vi "IO参数设置.vi"(8 "布尔文本.文本":string, 9 "section (optional)":string, 10 "监测项描述":string) -> (2 "增加？":bool, 3 "簇1输出":T1)   [LabVIEW 2016, in "环境动力监测库.lvlib"]
uses:
  <vilib>/Utility/miscctls.llb/LVPointTypeDef.ctl
  <vilib>/Utility/config.llb/NI_LVConfig.lvlib
panel:
  in  "模拟量配置":bool
  in  "传感器型号:":enum16{"PLC", "ZLAN"}(ring)
  in  "簇1输入":T1
  in  "返回":bool
  in  "增加":bool
  in  "告警参数:":enum32{"禁用告警", "闭合告警", "断开告警"}(radio)
  in  "端口:":T2(ring)
  in  "监测项描述:":string
  # "基本设置"
  # "如:红外XX"
  # "传感器选择"
  # "端口选择"
  # "参数设置"
  # "告警方式选择"
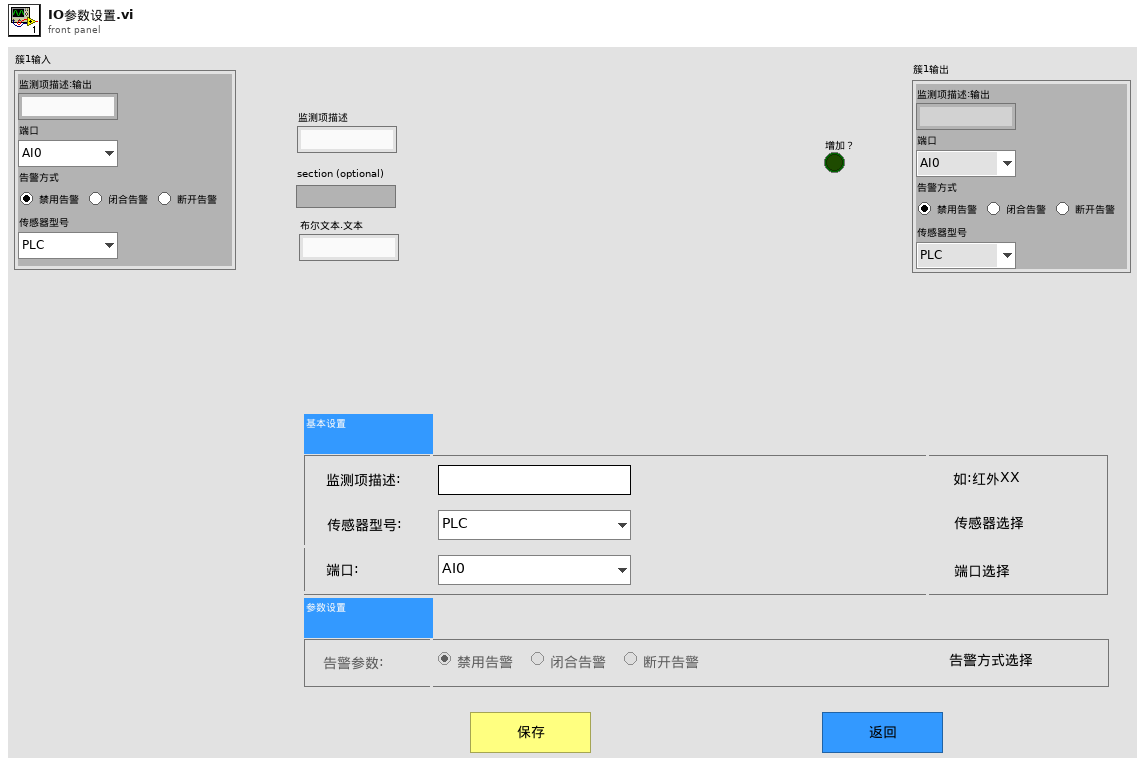
[diagram p1: front panel]
types:
  T1 = cluster{"监测项描述:输出":string, "端口":enum16{"AI0", "AI1", "AI2", "AI3", "AI4", "DI0", "DI1", "DI2", "DI3", "DI4", "DO0", "DO1", "DO2", "DO3", "DO4", "X0", "X1", "X2", "X3", "X4", "X5", "X6", "X7", "X8", "X9"}, "告警方式":enum32{"禁用告警", "闭合告警", "断开告警"}, "传感器型号":enum16{"PLC", "ZLAN"}}
  T2 = enum16{"AI0", "AI1", "AI2", "AI3", "AI4", "DI0", "DI1", "DI2", "DI3", "DI4", "DO0", "DO1", "DO2", "DO3", "DO4", "X0", "X1", "X2", "X3", "X4", "X5", "X6", "X7", "X8", "X9"}
  T3 = cluster{"模板选择:":enum16{"定时简报", "无(不告警)", "通用声光告警", "通用语言告警", "通用短信告警", "通用电话告警", "通用邮件告警", "通用声光+语音+短信告警", "通用声光+短信+电话告警", "通用多方式告警", "通用全方式告警", "自动按类型", "非告警时段", "自定义"}, "预警保持时间\n(s):":i16, "重复告警时间\n(s):":i16, "告警发送方式:":cluster{"声光":bool, "语音":bool, "短信":bool, "彩信":bool, "电话":bool, "邮件":bool, "联动1":bool, "联动2":bool}, "告警时段选择:":enum16{"全时段告警", "工作日告警", "周六周日告警", "非告警时段", "自定义"}, "告警抓拍设置:":enum16{"无"}, "告警短信内容:":string, "告警电话内容:":string, "告警解除方式:":cluster{"声光":bool, "语音":bool, "短信":bool, "彩信":bool, "电话":bool, "邮件":bool, "联动1":bool, "联动2":bool}, "告警解除内容:":string, "信息接收人:":cluster{"管理员":bool, "普通用户":bool}}
  T4 = typedef "LVPointTypeDef.ctl" = cluster{"Horizontal":i16, "Vertical":i16}
  T5 = typedef "NI_LVConfig.lvlib/Config Data RefNum.ctl" = refnum<k1>
  T6 = enum8{"Enabled", "Disabled", "Disabled and Grayed Out"}
  T7 = cluster{"漏水监测配置":cluster{"监测项描述:输出":string, "端口:":enum16{"AI0", "AI1", "AI2", "AI3", "AI4", "DI0", "DI1", "DI2", "DI3", "DI4", "DO0", "DO1", "DO2", "DO3", "DO4", "X0", "X1", "X2", "X3", "X4", "X5", "X6", "X7", "X8", "X9"}, "告警参数:":enum32{"禁用告警", "闭合告警", "断开告警"}, "传感器型号:":enum16{"PLC", "ZLAN"}}, "门禁开关监测配置":cluster{"监测项描述:输出":string, "端口:":enum16{"AI0", "AI1", "AI2", "AI3", "AI4", "DI0", "DI1", "DI2", "DI3", "DI4", "DO0", "DO1", "DO2", "DO3", "DO4", "X0", "X1", "X2", "X3", "X4", "X5", "X6", "X7", "X8", "X9"}, "告警参数:":enum32{"禁用告警", "闭合告警", "断开告警"}, "传感器型号:":enum16{"PLC", "ZLAN"}}, "温湿度监测配置":cluster{"监测项描述:输出":string, "端口:":enum16{"AI0", "AI1", "AI2", "AI3", "AI4", "DI0", "DI1", "DI2", "DI3", "DI4", "DO0", "DO1", "DO2", "DO3", "DO4", "X0", "X1", "X2", "X3", "X4", "X5", "X6", "X7", "X8", "X9"}, "告警参数:":enum32{"禁用告警", "闭合告警", "断开告警"}, "传感器型号:":enum16{"PLC", "ZLAN"}}, "烟雾监测配置":cluster{"监测项描述:输出":string, "端口:":enum16{"AI0", "AI1", "AI2", "AI3", "AI4", "DI0", "DI1", "DI2", "DI3", "DI4", "DO0", "DO1", "DO2", "DO3", "DO4", "X0", "X1", "X2", "X3", "X4", "X5", "X6", "X7", "X8", "X9"}, "告警参数:":enum32{"禁用告警", "闭合告警", "断开告警"}, "传感器型号:":enum16{"PLC", "ZLAN"}}, "冰箱监测配置":cluster{"监测项描述:输出":string, "端口:":enum16{"AI0", "AI1", "AI2", "AI3", "AI4", "DI0", "DI1", "DI2", "DI3", "DI4", "DO0", "DO1", "DO2", "DO3", "DO4", "X0", "X1", "X2", "X3", "X4", "X5", "X6", "X7", "X8", "X9"}, "告警参数:":enum32{"禁用告警", "闭合告警", "断开告警"}, "传感器型号:":enum16{"PLC", "ZLAN"}}, "排气扇监测配置":cluster{"监测项描述:输出":string, "端口:":enum16{"AI0", "AI1", "AI2", "AI3", "AI4", "DI0", "DI1", "DI2", "DI3", "DI4", "DO0", "DO1", "DO2", "DO3", "DO4", "X0", "X1", "X2", "X3", "X4", "X5", "X6", "X7", "X8", "X9"}, "告警参数:":enum32{"禁用告警", "闭合告警", "断开告警"}, "传感器型号:":enum16{"PLC", "ZLAN"}}}
  T8 = cluster{"原始值最小值":dbl, "原始值最大值":dbl, "转换值最小值":dbl, "转换值最大值":dbl, "原始值最小值 2":dbl, "原始值最大值 2":dbl, "转换值最小值 2":dbl, "转换值最大值 2":dbl, "原始值最小值 3":dbl, "原始值最大值 3":dbl, "转换值最小值 3":dbl, "转换值最大值 3":dbl, "原始值最小值 4":dbl, "原始值最大值 4":dbl, "转换值最小值 4":dbl, "转换值最大值 4":dbl, "转换值最大值 5":dbl, "转换值最小值 5":dbl, "原始值最大值 5":dbl, "原始值最小值 5":dbl, "转换值最大值 6":dbl, "转换值最小值 6":dbl, "原始值最大值 6":dbl, "原始值最小值 6":dbl, "转换值最大值 7":dbl, "转换值最小值 7":dbl, "原始值最大值 7":dbl, "原始值最小值 7":dbl, "转换值最大值 8":dbl, "转换值最小值 8":dbl, "原始值最大值 8":dbl, "原始值最小值 8":dbl}
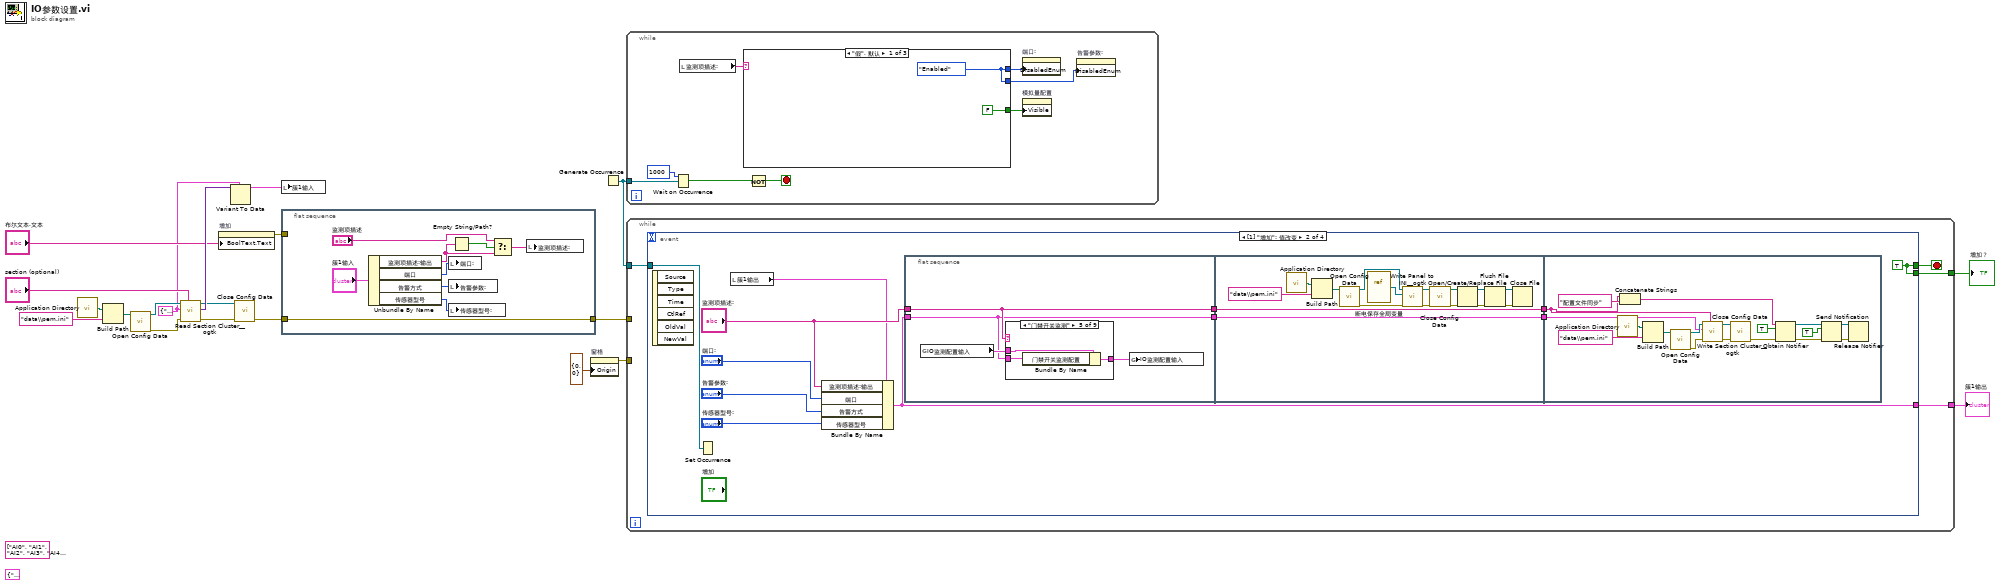
[diagram p0: block diagram]
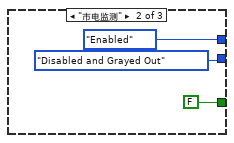
[diagram p2: hidden frame]
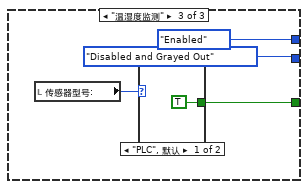
[diagram p3: hidden frame]
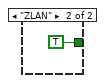
[diagram p4: hidden frame]
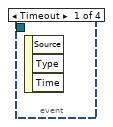
[diagram p5: hidden frame]
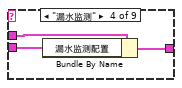
[diagram p9: hidden frame]
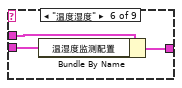
[diagram p10: hidden frame]
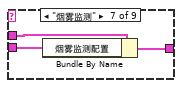
[diagram p11: hidden frame]
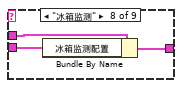
[diagram p12: hidden frame]
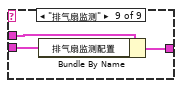
[diagram p13: hidden frame]
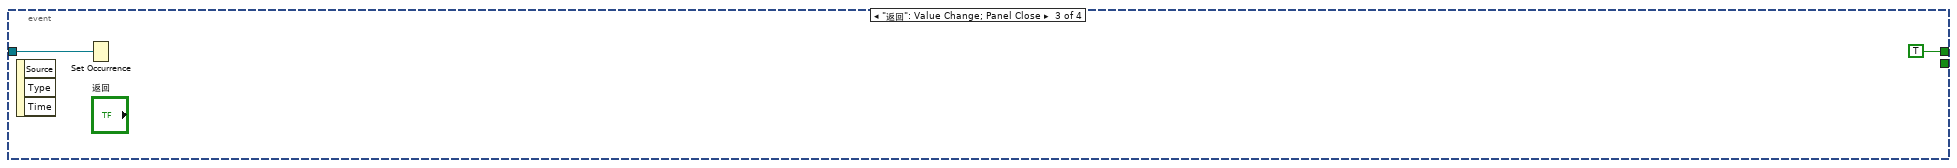
[diagram p14: hidden frame]
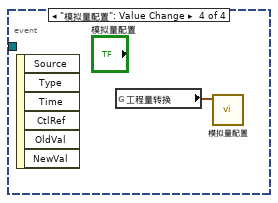
[diagram p15: hidden frame]
diagram:
  w1 = T1 {"监测项描述:输出"="", "端口"=enum."AI0", "告警方式"=enum."闭合告警", "传感器型号"=enum."PLC"} ("簇1输入")
  (unwired) string[] ["AI0", "AI1", "AI2", "AI3", "AI4", "DI0", "DI1", "DI2", "DI3", "DI4", "DO0", "DO1", "DO2", "DO3", "DO4", "X0", "X1", "X2", "X3", "X4", "X5", "X6", "X7", "X8", "X9"] ("字符串[]")
  (unwired) T3 {"模板选择:"=enum."定时简报", "预警保持时间\n(s):"=0, "重复告警时间\n(s):"=0, "告警发送方式:"={"声光"=FALSE, "语音"=FALSE, "短信"=FALSE, "彩信"=FALSE, "电话"=FALSE, "邮件"=FALSE, "联动1"=FALSE, "联动2"=FALSE}, "告警时段选择:"=enum."全时段告警", "告警抓拍设置:"=enum."无", "告警短信内容:"="", "告警电话内容:"="", "告警解除方式:"={"声光"=FALSE, "语音"=FALSE, "短信"=FALSE, "彩信"=FALSE, "电话"=FALSE, "邮件"=FALSE, "联动1"=FALSE, "联动2"=FALSE}, "告警解除内容:"="", "信息接收人:"={"管理员"=FALSE, "普通用户"=FALSE}} ("数据")
  n1 = call <vilib>:"Application Directory.vi"() -> ("Application Directory"=w14:path)
  n2 = Build Path(base path=w14, name or relative path="data\\pem.ini" ("名称或相对路径")) -> (appended path=w15:path)
  n3 = call <vilib>:"Open Config Data.vi"("configuration file path"=w15) -> ("error out"=w16:errorcluster, "refnum"=w17:T5)  [unwired: 8 in, 1 out]
  n4 = call <userlib>:"Read Section Cluster__ogtk.vi"("section (optional)"="section (optional)", "error in (no error)"=w16, "Section Formatted Cluster Type"=w1, "refnum"=w17) -> ("error out"=w4:errorcluster, "Section Formatted Cluster"=w11:variant, "dup refnum"=w5:T5)  [unwired: 3 in, 2 out]
  n5 = property on="增加" class="Bool"("BoolText.Text"="布尔文本.文本") -> (error out=w7:errorcluster)  [unwired: 2 in, 1 out]
  n6 = Variant To Data(type=w1, Variant=w11) -> (data=w6:T1)  [unwired: 1 in, 1 out]
  n7 = call <vilib>:"Close Config Data.vi"("error in (no error)"=w4, "refnum"=w5) -> ("error out"=w10:errorcluster)  [unwired: 8 in, 1 out]
  n8 = local write "簇1输入"(w6) -> ()
  n9 = flat-sequence {
    tunnel: w10 -> [w28]
    tunnel: [w28] -> w9
    tunnel: w7 -> [_]
    frame #0 {
      n10 = Unbundle By Name("簇1输入") -> ("监测项描述:输出"=w25:string, "端口"=w23:T2, "告警方式"=w22:enum32{"禁用告警", "闭合告警", "断开告警"}, "传感器型号"=w21:enum16{"PLC", "ZLAN"})
      n11 = local write "端口:"(w23) -> ()
      n12 = local write "告警参数:"(w22) -> ()
      n13 = local write "传感器型号:"(w21) -> ()
      n14 = Empty String/Path?(string/path=w25) -> (empty?=w27:bool)
      n15 = Select(t="监测项描述", s=w27, f=w25) -> (s? t:f=w24:string)
      n16 = local write "监测项描述:"(w24) -> ()
    }
  }
  n17 = property on="窗格" class="Pane"("Origin"=T4 {"Horizontal"=0, "Vertical"=0} ("原点")) -> (error out=w18:errorcluster)  [unwired: 2 in, 1 out]
  n18 = Generate Occurrence() -> (w3:refnum<k4>)
  n19 = while {
    tunnel: w3 -> [w35]
    stop <- w34 stop-if-true
    n20 = Wait on Occurrence(2:w35, 3:1000 ("毫秒超时(-1)")) -> (0:w36:bool)  [unwired: 1 in]
    n21 = local read "监测项描述:"() -> (w33:string)
    n22 = case shown="\"假\", 默认" w33 {
      tunnel: [FALSE ("可见") FALSE ("可见") w45] -> w32
      tunnel: [w38 T6."Enabled" ("禁用") T6."Enabled" ("禁用")] -> w31
      tunnel: [w38 T6."Disabled and Grayed Out" ("禁用") T6."Disabled and Grayed Out" ("禁用")] -> w30
      frame "假", Default {
        w38 = T6."Enabled" ("禁用")
      }
      frame "市电监测" {
      }
      frame "温湿度监测" {
        n23 = local read "传感器型号:"() -> (w46:enum16{"PLC", "ZLAN"})
        n24 = case shown="\"PLC\", 默认" w46 {
          tunnel: [TRUE ("可见") TRUE ("可见")] -> w45
          frame "PLC", Default {
          }
          frame "ZLAN" {
          }
        }
      }
    }
    n25 = Not(x=w36) -> (.not. x?=w34:bool)
    n26 = property on="端口:" class="Enum (严格)"("DisabledEnum"=w31) -> ()  [unwired: 2 in, 2 out]
    n27 = property on="模拟量配置" class="Bool"("Visible"=w32) -> ()  [unwired: 2 in, 2 out]
    n28 = property on="告警参数:" class="RadioBtnsControl (严格)"("DisabledEnum"=w30) -> ()  [unwired: 2 in, 2 out]
  }
  n29 = while {
    tunnel: [w52] -> w2
    tunnel: [w50] -> w20
    tunnel: w18 -> [_]
    tunnel: w9 -> [_]
    tunnel: w3 -> [w49]
    stop <- w51 stop-if-true
    n30 = event shown="[1] \"增加\": 值改变" {
      selector: _ -> [_ _ _ _]
      dyn-events: _ -> [_ _ _ _]
      timeout: _ -> [_ _ _ _]
      tunnel: [_ w64 TRUE _] -> w51
      tunnel: [_ w57 _ _] -> w52
      tunnel: [_ w64 _ _] -> w50
      tunnel: w49 -> [_ w62 w124 _]
      event Timeout {
        n31 = event-data() -> ()  [unwired: 1 in, 3 out]
      }
      event "增加": Value Change {
        w64 = TRUE
        n32 = event-data() -> ()  [unwired: 1 in, 6 out]
        n33 = Set Occurrence(w62) -> ()
        n34 = local read "簇1输出"() -> (w61:T1)
        n35 = Bundle By Name(cluster=w61, "监测项描述:输出"="监测项描述:", "端口"="端口:", "告警方式"="告警参数:", "传感器型号"="传感器型号:") -> (w57:T1)
        n36 = flat-sequence {
          tunnel: "监测项描述:" -> [w66]
          tunnel: w57 -> [w65]
          tunnel: [w66] -> w56
          tunnel: [w65] -> w54
          tunnel: w56 -> [w91]
          tunnel: [w91] -> w55
          tunnel: w54 -> [w90]
          tunnel: [w90] -> w53
          tunnel: w55 -> [w107]
          tunnel: w53 -> [w109]
          frame #0 {
            n37 = global read "断电保存全局变量.vi" "IO监测配置输入"() -> (w68:T7)
            n38 = case shown="\"门禁开关监测\"" w66 {
              tunnel: w68 -> [w69 w70 w71 w74 w77 w80 w83 w86 w89]
              tunnel: [w69 w70 w71 w73 w76 w79 w82 w85 w88] -> w67
              tunnel: w65 -> [_ _ _ w72 w75 w78 w81 w84 w87]
              frame "假", Default {
              }
              frame "市电监测" {
              }
              frame "空调监测" {
              }
              frame "漏水监测" {
                n39 = Bundle By Name(cluster=w74, "漏水监测配置"=w72) -> (w73:T7)
              }
              frame "门禁开关监测" {
                n40 = Bundle By Name(cluster=w77, "门禁开关监测配置"=w75) -> (w76:T7)
              }
              frame "温度湿度" {
                n41 = Bundle By Name(cluster=w80, "温湿度监测配置"=w78) -> (w79:T7)
              }
              frame "烟雾监测" {
                n42 = Bundle By Name(cluster=w83, "烟雾监测配置"=w81) -> (w82:T7)
              }
              frame "冰箱监测" {
                n43 = Bundle By Name(cluster=w86, "冰箱监测配置"=w84) -> (w85:T7)
              }
              frame "排气扇监测" {
                n44 = Bundle By Name(cluster=w89, "排气扇监测配置"=w87) -> (w88:T7)
              }
            }
            n45 = global write "断电保存全局变量.vi" "IO监测配置输入"(w67) -> ()
          }
          frame #1 {
            n46 = call <vilib>:"Application Directory.vi"() -> ("Application Directory"=w105:path)
            n47 = Build Path(base path=w105, name or relative path="data\\pem.ini" ("名称或相对路径")) -> (appended path=w103:path)
            n48 = call <vilib>:"Open Config Data.vi"("configuration file path"=w103) -> ("error out"=w101:errorcluster, "refnum"=w102:T5)  [unwired: 8 in, 1 out]
            n49 = vi-ref "断电保存全局变量.vi"() -> (w92:refnum<vi>)
            n50 = call <userlib>:"Write Panel to INI__ogtk.vi"("error in (no error)"=w101, "VI ref"=w92, "refnum"=w102) -> ("error out"=w99:errorcluster, "refnum out"=w100:T5)  [unwired: 7 in]
            n51 = call <vilib>:"Close Config Data.vi"("error in (no error)"=w99, "refnum"=w100) -> ("error out"=w93:errorcluster, "file path"=w94:path)  [unwired: 8 in]
            n52 = Open/Create/Replace File(file path (use dialog)=w94, error in=w93) -> (refnum out=w97:refnum<file>, error out=w98:errorcluster)  [unwired: 4 in, 1 out]
            n53 = Flush File(refnum=w97, error in=w98) -> (refnum out=w96:refnum<file>, error out=w95:errorcluster)
            n54 = Close File(refnum=w96, error in=w95) -> ()  [unwired: 2 out]
          }
          frame #2 {
            n55 = call <vilib>:"Application Directory.vi"() -> ("Application Directory"=w112:path)
            n56 = Concatenate Strings(w107, "配置文件同步" ("名称（未命名）")) -> (w106:string)
            n57 = Build Path(base path=w112, name or relative path="data\\pem.ini" ("名称或相对路径")) -> (appended path=w111:path)
            n58 = call <vilib>:"Open Config Data.vi"("configuration file path"=w111) -> ("error out"=w110:errorcluster, "refnum"=w123:T5)  [unwired: 8 in, 1 out]
            n59 = call <userlib>:"Write Section Cluster__ogtk.vi"("section (optional)"=w107, "error in (no error)"=w110, "Section Formatted Cluster"=w109, "refnum"=w123) -> ("error out"=w122:errorcluster, "dup refnum"=w121:T5)  [unwired: 6 in]
            n60 = call <vilib>:"Close Config Data.vi"("error in (no error)"=w122, "refnum"=w121) -> ("error out"=w118:errorcluster)  [unwired: 8 in, 1 out]
            n61 = Obtain Notifier(name (unnamed)=w106, notification data type=TRUE, error in (no error)=w118) -> (notifier out=w116:refnum<notifier>, error out=w117:errorcluster)  [unwired: 1 in, 1 out]
            n62 = Send Notification(notification=TRUE ("通知"), notifier=w116, error in (no error)=w117) -> (notifier out=w119:refnum<notifier>, error out=w120:errorcluster)
            n63 = Release Notifier(notifier=w119, error in (no error)=w120) -> ()  [unwired: 1 in, 3 out]
          }
        }
      }
      event "返回": Value Change; Panel Close {
        n64 = event-data() -> ()  [unwired: 1 in, 3 out]
        n65 = Set Occurrence(w124) -> ()
      }
      event "模拟量配置": Value Change {
        n66 = event-data() -> ()  [unwired: 1 in, 6 out]
        n67 = global read "通讯全局变量断电保存.vi" "工程量转换"() -> (w126:T8)
        n68 = call "模拟量配置.vi"("工程量转换"=w126) -> ()  [unwired: 11 in]
      }
    }
  }
  "增加？" <- w20
  "簇1输出" <- w2
